vi "measure_dc2400_4wire_lxy.vi"(8 "error out":errorcluster, 11 "2400 resource name":refnum<visa-resource-name>) -> (0 "error out 2":errorcluster caption="错误输出 2", 2 "2400 resource name out":refnum<visa-resource-name>, 3 "输出数组":string[](array[string]))   [LabVIEW 2019, in "nematic.lvlib"]
uses:
  nematic.lvlib
  <vilib>/Analysis/baseanly.llb/Mean (DBL).vi
  lib/Keithley 24XX/Public/Data/Read (Single Point).vi
  lib/Keithley 24XX/Keithley 24XX.lvlib
  <vilib>/Analysis/NI_AALBase.lvlib
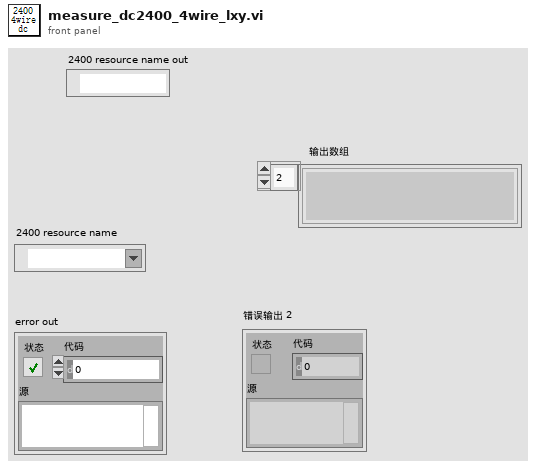
[diagram p1: front panel]
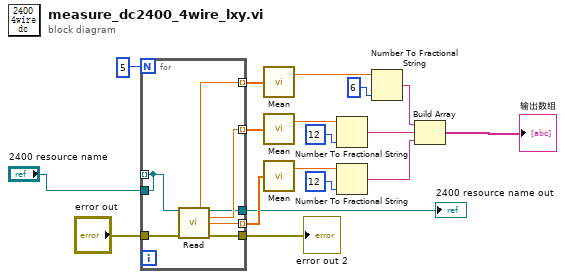
[diagram p0: block diagram]
diagram:
  n1 = for {
    N: 5 -> [_]
    tunnel: [w25] -> w17 mode=indexing
    tunnel: [w24] -> w16 mode=indexing
    tunnel: [w23] -> w15 mode=indexing
    tunnel: [w22] -> w3
    tunnel: [w19] -> _ mode=indexing
    tunnel: "error out" -> [w21]
    tunnel: [w20] -> w2
    tunnel: "2400 resource name" -> [w19]
    n2 = call-poly "Read.vi"("VISA resource name"=w19, "error in (no error)"=w21) -> ("Voltage"=w25:sgl, "VISA resource name out"=w20:refnum<visa-resource-name>, "Current"=w24:sgl, "Resistance"=w23:sgl, "error out"=w22:errorcluster)  [unwired: 7 in, 2 out]
  }
  "error out 2" <- w3
  "2400 resource name out" <- w2
  n3 = call-poly <vilib>:"Mean.vi"("X"=w17) -> ("mean"=w12:dbl)  [unwired: 1 out]
  n4 = call-poly <vilib>:"Mean.vi"("X"=w16) -> ("mean"=w14:dbl)  [unwired: 1 out]
  n5 = call-poly <vilib>:"Mean.vi"("X"=w15) -> ("mean"=w13:dbl)  [unwired: 1 out]
  n6 = Number To Fractional String(number=w14, precision (6)=i16 12 ("精度(6)")) -> (F-format string=w7:string)  [unwired: 2 in]
  n7 = Number To Fractional String(number=w13, precision (6)=i16 12 ("精度(6)")) -> (F-format string=w6:string)  [unwired: 2 in]
  n8 = Number To Fractional String(number=w12, precision (6)=i16 6 ("精度(6)")) -> (F-format string=w8:string)  [unwired: 2 in]
  n9 = Build Array(w8, w7, w6) -> (→"输出数组":string[])
